vi "Set_Channel_Map.vi"() -> ()   [LabVIEW 2021]
uses:
  Channel_Cluster.ctl
  Channel_Map_Global.vi
panel:
  out "Channels map":T1[](array[typedef])
  in  "Reset map":bool
  in  "End configuration":bool
  in  "Remove channel":bool
  in  "Add channel":bool
  in  "Channel":u8=2 min=2 max=13 step=1
  in  "Channel name":string
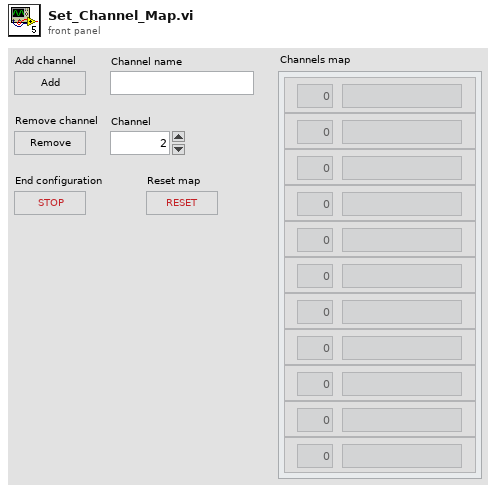
[diagram p1: front panel]
types:
  T1 = typedef "Channel_Cluster.ctl" = cluster{"Channel name":string, "Channel":u8}
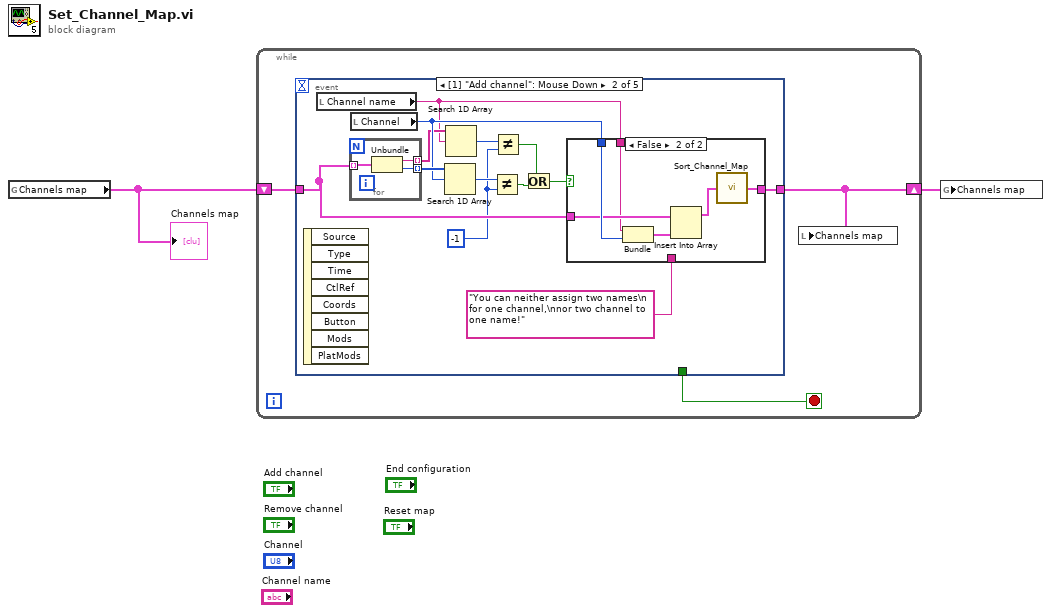
[diagram p0: block diagram]
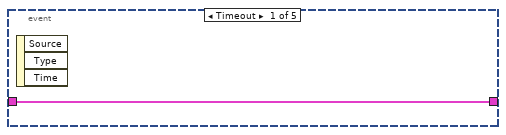
[diagram p2: hidden frame]
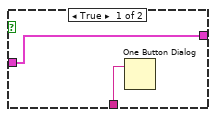
[diagram p3: hidden frame]
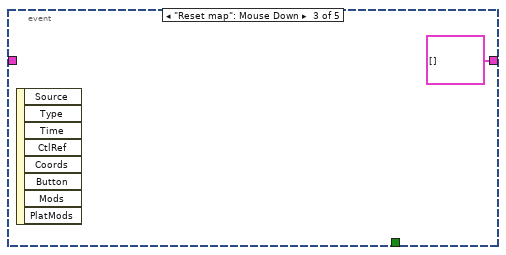
[diagram p4: hidden frame]
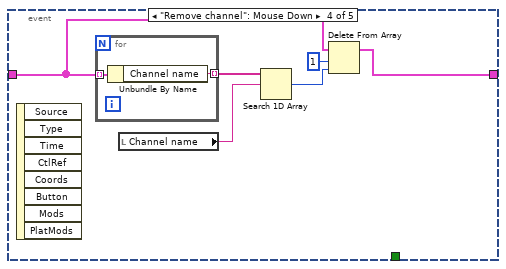
[diagram p5: hidden frame]
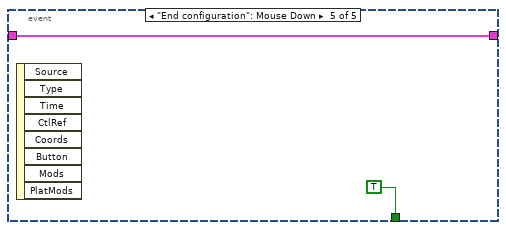
[diagram p6: hidden frame]
diagram:
  n1 = global read "Channel_Map_Global.vi" "Channels map"() -> (w1:T1[])
  "Channels map" <- w1
  n2 = while {
    shift-right: [w3] -> w2
    shift-left: w1 -> [w5]
    stop <- w4 stop-if-true
    n3 = event shown="[1] \"Add channel\": Mouse Down" {
      selector: _ -> [_ _ _ _ _]
      dyn-events: _ -> [_ _ _ _ _]
      timeout: _ -> [_ _ _ _ _]
      tunnel: w5 -> [w6 w18 _ w35 w41]
      tunnel: [w6 w15 T1[] [] w32 w41] -> w3
      tunnel: [_ _ _ _ TRUE] -> w4
      event Timeout {
        n4 = event-data() -> ()  [unwired: 1 in, 3 out]
      }
      event "Add channel": Mouse Down {
        w11 = -1 ("y")
        n5 = event-data() -> ()  [unwired: 1 in, 8 out]
        n6 = local read "Channel name"() -> (w7:string)
        n7 = for {
          tunnel: w18 -> [w30] mode=indexing
          tunnel: [w29] -> w19 mode=indexing
          tunnel: [w28] -> w13 mode=indexing
          n8 = Unbundle(w30) -> ("Channel name"=w28:string, "Channel"=w29:u8)
        }
        n9 = local read "Channel"() -> (w17:u8)
        n10 = Search 1D Array(1D array=w19, element=w17) -> (index of element=w14:i32)  [unwired: 1 in]
        n11 = Search 1D Array(1D array=w13, element=w7) -> (index of element=w12:i32)  [unwired: 1 in]
        n12 = Not Equal?(x=w14, y=w11) -> (x != y?=w9:bool)
        n13 = Not Equal?(x=w12, y=w11) -> (x != y?=w10:bool)
        n14 = Or(x=w10, y=w9) -> (x .or. y?=w8:bool)
        n15 = case shown="False" w8 {
          tunnel: [w20 w24] -> w15
          tunnel: w18 -> [w20 w26]
          tunnel: w17 -> [_ w27]
          tunnel: "You can neither assign two names\n for one channel,\nnor two channel to one name!" ("message") -> [w21 _]
          tunnel: w7 -> [_ w22]
          frame True {
            n16 = One Button Dialog(message=w21) -> ()  [unwired: 1 in, 1 out]
          }
          frame False {
            n17 = Bundle("Channel name"=w22, "Channel"=w27) -> (w25:cluster{"Channel name":string, "Channel":u8})  [unwired: 1 in]
            n18 = Insert Into Array(array=w26, new element=w25) -> (w23:T1[])  [unwired: 1 in]
            n19 = call "Sort_Channel_Map.vi"("Channels map"=w23) -> ("Sorted Channels map"=w24:T1[])
          }
        }
      }
      event "Reset map": Mouse Down {
        n20 = event-data() -> ()  [unwired: 1 in, 8 out]
      }
      event "Remove channel": Mouse Down {
        n21 = event-data() -> ()  [unwired: 1 in, 8 out]
        n22 = for {
          tunnel: w35 -> [w39] mode=indexing
          tunnel: [w38] -> w37 mode=indexing
          n23 = Unbundle By Name(w39) -> ("Channel name"=w38:string)
        }
        n24 = local read "Channel name"() -> (w36:string)
        n25 = Search 1D Array(1D array=w37, element=w36) -> (index of element=w33:i32)  [unwired: 1 in]
        n26 = Delete From Array(array=w35, length=1, index=w33) -> (array with subset deleted=w32:T1[])  [unwired: 1 out]
      }
      event "End configuration": Mouse Down {
        n27 = event-data() -> ()  [unwired: 1 in, 8 out]
      }
    }
    n28 = local write "Channels map"(w3) -> ()
  }
  n29 = global write "Channel_Map_Global.vi" "Channels map"(w2) -> ()
